vi "CLC_Gen3_L1_ComGainPhase_ENA.vi"() -> ()   [LabVIEW 2023, in "Clover_Cell.lvlib"]
uses:
  lib/CTL/Keysight_VNA.ctl
  Clover_Cell.lvlib
  lib/Keysight/Keysight.lvlib
panel:
  in  "Element Gain":i32
  in  "Waiting Time(ms)":u32=100
  in  "sParameter":i32=21
  in  "Step_Freq(GHz)":dbl=0.5 format="%#_13g"
  in  "Stop_Freq(GHz)":dbl=31.5
  in  "Start_Freq(GHz)":dbl=26.5
  in  "Polarity":u16(ring) items=["H", "V"]
  in  "TRXmode":u16(ring)=1 items=["Rx"=2, "Tx"=1]
  out "Step-2":bool
  out "PHASE 2":i32
  out "GAIN 2":i32
  out "Channel 2":i32
  out "Step-1":bool
  out "Channel":i32
  out "GAIN":i32
  out "PHASE":i32
  out "Marker_array":dbl[](array[numeric])
  out "Phase":dbl[][](graph)
  in  "FileName_Note":string
  in  "VISA resource name":refnum<visa-resource-name>="TCPIP0::192.168.100.12::inst0::INSTR"
  out "Return State":bool
  out "output cluster":T1={"address"="192.168.100.111", "remote port or service name"=5025, "timeout ms (60000)"=10000}
  out "Gain":dbl[][](graph)
  out "error out":errorcluster
  # "CLC-Gen3-L1-COMGainPhase-Sweep-ENA"
  # "Setting"
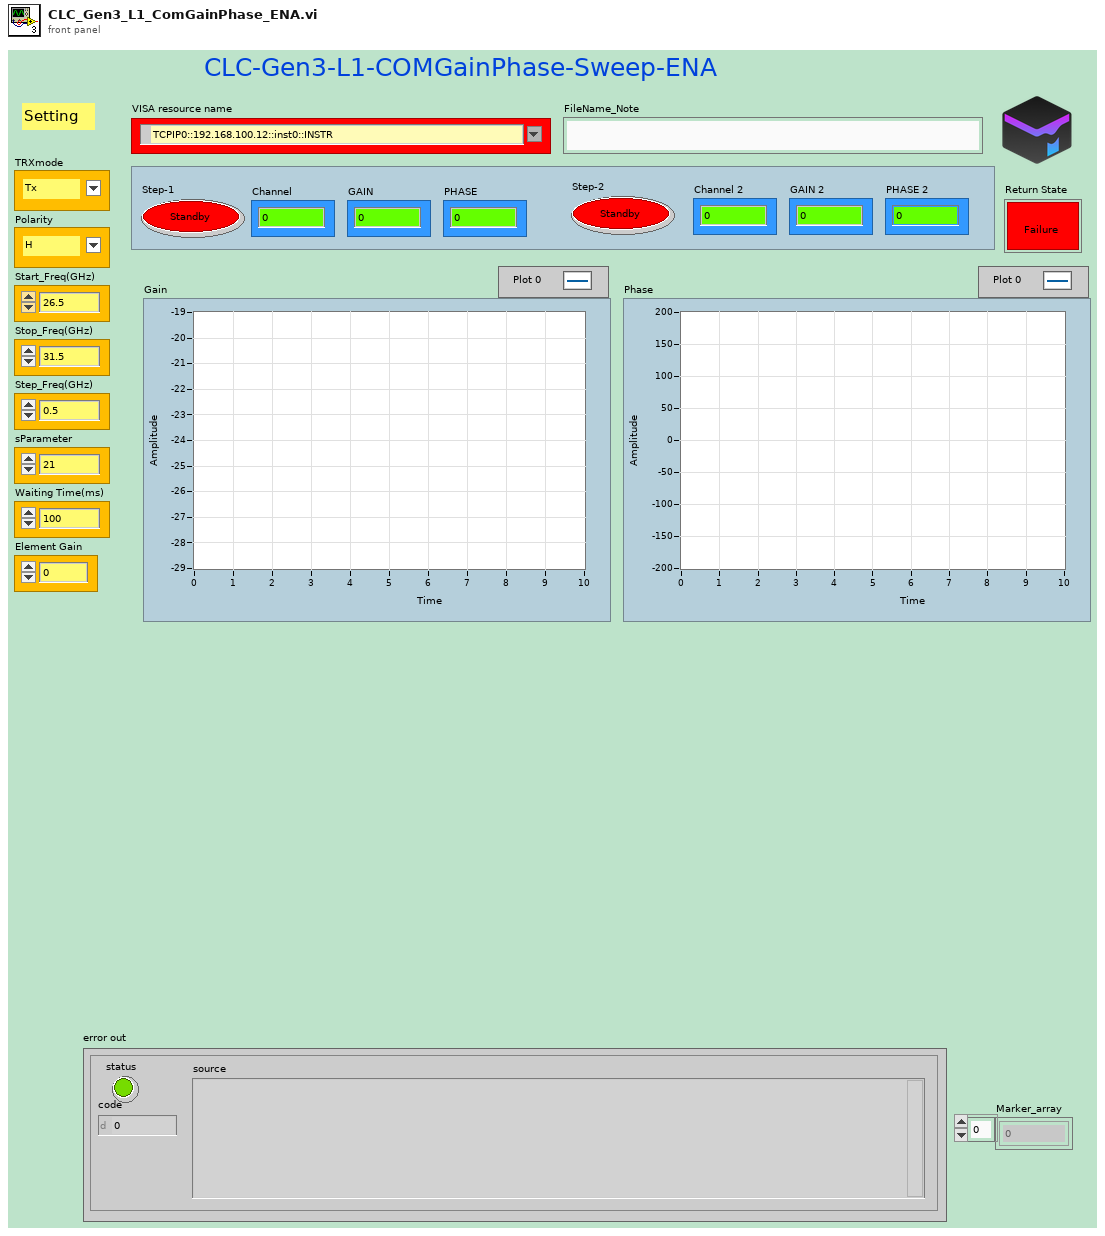
[diagram p1: front panel]
types:
  T1 = cluster{"address":string, "remote port or service name":u16, "timeout ms (60000)":i32}
  T2 = typedef "Keysight_VNA.ctl" = enum16{"Init", "queryMarker", "setSweepPoint", "setMarkerFreq", "setMeasureFormat", "setFreqStartStop", "setMarkerOnOFF", "setMarkerFormat_LOGP", "setMeasPAR_S", "setTriggerSingle", "Trigger_Save_SnP", "Trigger_Single", "Close"}
  T3 = cluster{"Mode":u16, "Polarity":u16, "CH_ON/OFF":u16, "Channel":i32, "Gain":i32, "Phase":i32}
  T4 = cluster{"setSweepPoint":i32, "Meas":i32, "Mark":i32, "Freq_GHz":dbl, "Start_Freq(GHz)":dbl, "Stop_Freq(GHz)":dbl, "sParameter":i32}
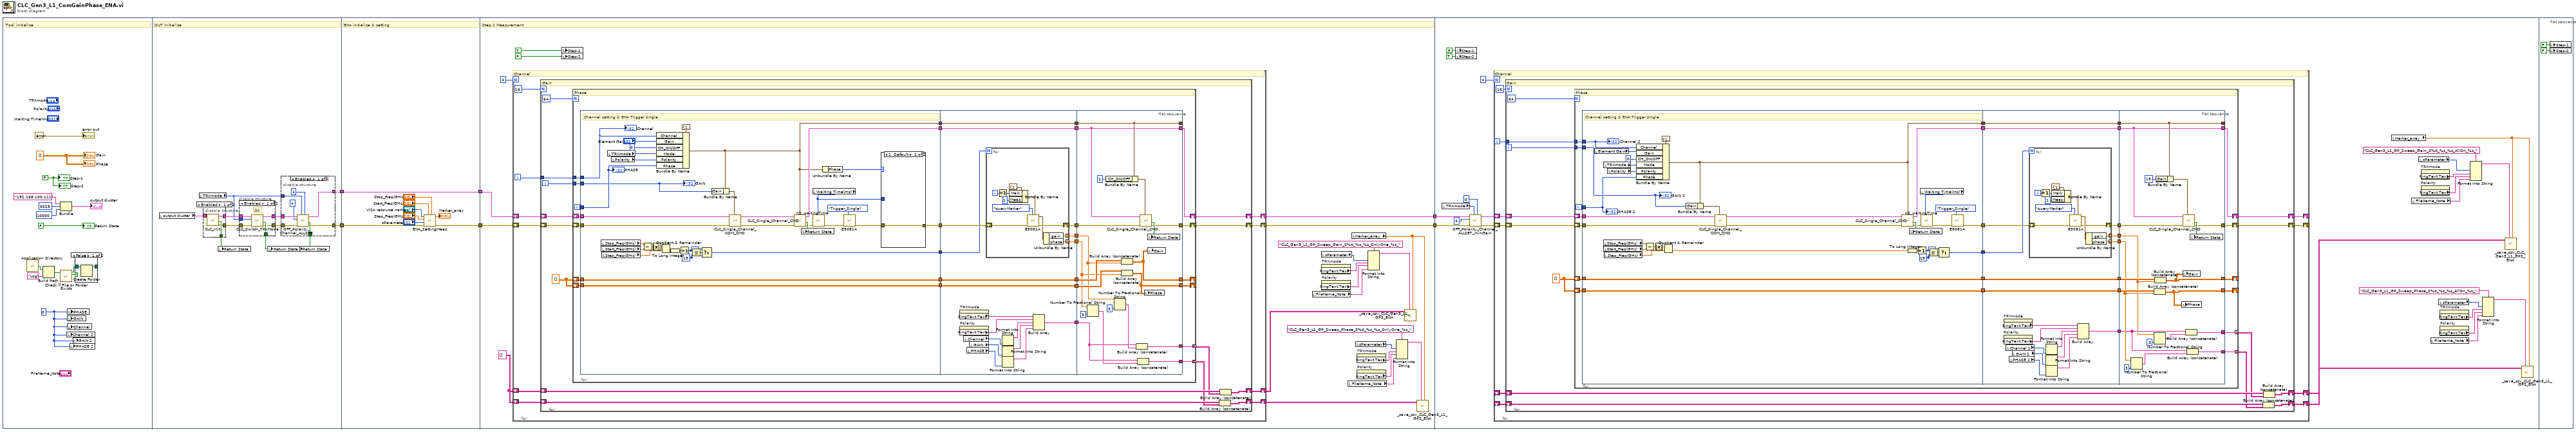
[diagram p0: block diagram]
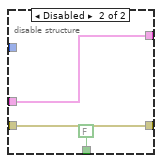
[diagram p3: hidden frame]
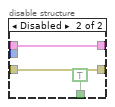
[diagram p4: hidden frame]
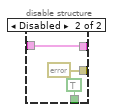
[diagram p5: hidden frame]
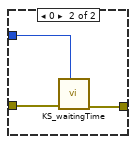
[diagram p6: hidden frame]
diagram:
  n1 = flat-sequence {
    tunnel: [w25] -> w6
    tunnel: [w29] -> w5
    tunnel: w6 -> [w70]
    tunnel: w5 -> [w63]
    tunnel: [w70] -> w4
    tunnel: [w64] -> w3
    tunnel: w4 -> [w93]
    tunnel: w3 -> [w90]
    tunnel: [w92] -> w2
    tunnel: [w91] -> w1
    tunnel: w2 -> [w254]
    tunnel: w1 -> [w255]
    frame #0 {
      w8 = FALSE ("Step-1")
      w7 = 0 ("PHASE")
      w9 = dbl[][] []
      # "Tool initialize"
      n2 = call <vilib>:"Application Directory.vi"() -> ("Application Directory"=w13:path)
      n3 = Build Path(base path=w13, name or relative path="Log") -> (appended path=w10:path)
      n4 = Bundle("address"="192.168.100.111", "remote port or service name"=u16 5025, "timeout ms (60000)"=10000) -> (→"output cluster":T1)  [unwired: 1 in]
      n5 = call <vilib>:"Check if File or Folder Exists.vi"("path"=w10) -> ("file or folder exists?"=w12:bool, "dup path"=w11:path)  [unwired: 8 in, 1 out]
      n6 = local write "Channel 2"(w7) -> ()
      n7 = local write "PHASE"(w7) -> ()
      n8 = local write "GAIN"(w7) -> ()
      n9 = local write "Channel"(w7) -> ()
      n10 = local write "PHASE 2"(w7) -> ()
      n11 = local write "GAIN 2"(w7) -> ()
      n12 = case shown="False" w12 {
        tunnel: w11 -> [w22 w23]
        tunnel: [w21 w23] -> _
        frame False {
          n13 = Create Folder(path (use dialog)=w22) -> (created path=w21:path)  [unwired: 2 in, 2 out]
        }
        frame True {
        }
      }
      "error out" <- errorcluster {"status"=FALSE, "code"=0, "source"=""} ("error out")
      "Return State" <- FALSE ("OK?")
      "Gain" <- w9
      "Phase" <- w9
      "Step-1" <- w8
      "Step-2" <- w8
    }
    frame #1 {
      # "DUT initialize"
      n14 = local read "output cluster"() -> (w34:T1)
      n15 = local read "TRXmode"() -> (w24:u16)
      n16 = disable-structure shown="Enabled" {
        disable-tunnel: w34 -> [w58 w61]
        disable-tunnel: [w57 w61] -> w33
        disable-tunnel: [w56 errorcluster {"status"=FALSE, "code"=0, "source"=""} ("error in (no error)")] -> w31
        disable-tunnel: [w55 TRUE ("OK?")] -> w26
        frame Enabled {
          n17 = call "CLC_Init.vi"("TCPIPin"=w58) -> ("error out"=w56:errorcluster, "Status"=w55:bool, "TCPIPin 2"=w57:T1)  [unwired: 8 in]
        }
        frame Disabled {
        }
      }
      n18 = local write "Return State"(w26) -> ()
      n19 = disable-structure shown="Enabled" {
        disable-tunnel: w33 -> [w51 w53]
        disable-tunnel: [w50 TRUE ("OK?")] -> w32
        disable-tunnel: w31 -> [w49 w52]
        disable-tunnel: [w48 w52] -> w30
        disable-tunnel: [w47 w53] -> w28
        disable-tunnel: w24 -> [w46 _]
        frame Enabled {
          # "OK"
          n20 = call "CLC_Switch_TRxMode.vi"("error in (no error)"=w49, "Text Ring"=w46, "TCPIPin"=w51) -> ("error out"=w48:errorcluster, "OK?"=w50:bool, "TCPIPin 2"=w47:T1)  [unwired: 6 in]
        }
        frame Disabled {
        }
      }
      n21 = local write "Return State"(w32) -> ()
      n22 = disable-structure shown="Enabled" {
        disable-tunnel: w30 -> [w42 w44]
        disable-tunnel: [w41 w44] -> w29
        disable-tunnel: w28 -> [w40 w43]
        disable-tunnel: [w39 FALSE ("OK?")] -> w27
        disable-tunnel: w24 -> [w37 _]
        disable-tunnel: [w35 w43] -> w25
        frame Enabled {
          n23 = call "OFF_Polarity_Channel_ALLSET.vi"("CH_ON:0/OFF:1"=u16 1, "Mode"=w37, "error in"=w42, "Channel"=4, "TCPIPin"=w40) -> ("error out"=w41:errorcluster, "OK?"=w39:bool, "TCPIPout"=w35:T1)  [unwired: 4 in]
        }
        frame Disabled {
        }
      }
      n24 = local write "Return State"(w27) -> ()
    }
    frame #2 {
      # "ENA initialize & setting"
      n25 = call "ENA_SettingMeas.vi"("Stop_Freq(GHz)"="Stop_Freq(GHz)", "Start_Freq(GHz)"="Start_Freq(GHz)", "error in"=w63, "sParameter"="sParameter", "Step_Freq(GHz)"="Step_Freq(GHz)", "VISA IN"="VISA resource name") -> ("error out"=w64:errorcluster, "Marker_array"=→"Marker_array":dbl[])  [unwired: 4 in]
    }
    frame #3 {
      w88 = string[][] []
      # "Step.1 Measurement"
      n26 = for {
        N: 4 -> [_]
        shift-right: [w102] -> w92
        shift-left: w93 -> [w103]
        shift-right: [w101] -> w91
        shift-left: w90 -> [w100]
        shift-right: [w95] -> w87
        shift-left: w88 -> [w97]
        shift-right: [w94] -> w86
        shift-left: w88 -> [w96]
        i -> [w98]
        # "Channel"
        n27 = for {
          N: 16 -> [_]
          shift-right: [w116] -> w102
          shift-left: w103 -> [w117]
          shift-right: [w115] -> w101
          shift-left: w100 -> [w114]
          tunnel: w98 -> [w112]
          shift-right: [w106] -> w95
          shift-left: w97 -> [w110]
          shift-right: [w105] -> w94
          shift-left: w96 -> [w109]
          i -> [w111]
          w104 = dbl[][] []
          # "Gain"
          n28 = for {
            N: 64 -> [_]
            shift-right: [w132] -> w116
            shift-left: w117 -> [w144]
            shift-right: [w131] -> w115
            shift-left: w114 -> [w143]
            tunnel: w112 -> [w142]
            tunnel: w111 -> [w141]
            tunnel: [w127] -> w108 mode=indexing
            tunnel: [w126] -> w107 mode=indexing
            shift-right: [w119] -> _
            shift-left: w104 -> [w123]
            shift-right: [w118] -> _
            shift-left: w104 -> [w120]
            i -> [w140]
            # "Phase"
            n29 = flat-sequence {
              tunnel: w144 -> [w154]
              tunnel: w143 -> [w155]
              tunnel: w142 -> [w178]
              tunnel: w141 -> [w151]
              tunnel: w140 -> [w171]
              tunnel: [w148] -> w139
              tunnel: [w160] -> w138
              tunnel: [w146] -> w137
              tunnel: [w159] -> w136
              tunnel: [w158] -> w124
              tunnel: w123 -> [w158]
              tunnel: [w157] -> w121
              tunnel: w120 -> [w157]
              tunnel: w139 -> [w201]
              tunnel: w138 -> [w200]
              tunnel: w137 -> [w199]
              tunnel: w136 -> [w198]
              tunnel: [w202] -> w135
              tunnel: [w200] -> w134
              tunnel: [w199] -> w133
              tunnel: [w197] -> w130
              tunnel: [w196] -> w129
              tunnel: [w187] -> w128
              tunnel: [w186] -> w125
              tunnel: w124 -> [w186]
              tunnel: [w185] -> w122
              tunnel: w121 -> [w185]
              tunnel: [w230] -> _
              tunnel: [w227] -> w132
              tunnel: [w232] -> w131
              tunnel: w135 -> [w231]
              tunnel: w134 -> [w227]
              tunnel: w133 -> [w230]
              tunnel: w130 -> [w217]
              tunnel: w129 -> [w216]
              tunnel: w128 -> [w223]
              tunnel: [w221] -> w127
              tunnel: [w220] -> w126
              tunnel: w125 -> [w219]
              tunnel: w122 -> [w218]
              tunnel: [w215] -> w119
              tunnel: [w214] -> w118
              frame #0 {
                w170 = 15 ("y")
                # "Channel setting & ENA Trigger single"
                n30 = local read "Stop_Freq(GHz)"() -> (w163:dbl)
                n31 = local read "Start_Freq(GHz)"() -> (w162:dbl)
                n32 = local read "Step_Freq(GHz)"() -> (w161:dbl)
                n33 = local read "TRXmode"() -> (w176:u16)
                n34 = local read "Polarity"() -> (w177:u16)
                n35 = Subtract(x=w163, y=w162) -> (x-y=w169:dbl)
                n36 = Absolute Value(x=w169) -> (abs(x)=w168:dbl)
                n37 = Bundle By Name(cluster=T3 {"Mode"=1, "Polarity"=1, "CH_ON/OFF"=1, "Channel"=0, "Gain"=0, "Phase"=0} ("Channel params"), "Channel"=w178, "Gain"="Element Gain", "CH_ON/OFF"=u16 0, "Mode"=w176, "Polarity"=w177, "Phase"=w171) -> (w146:T3)
                n38 = Quotient & Remainder(x=w168, y=w161) -> (floor(x/y)=w167:dbl)  [unwired: 1 out]
                n39 = To Long Integer(number=w167) -> (32bit integer=w166:i32)
                n40 = Increment(x=w166) -> (x+1=w164:i32)
                n41 = Less Or Equal?(x=w164, y=w170) -> (x <= y?=w165:bool)
                n42 = Select(t=w164, s=w165, f=w170) -> (s? t:f=w159:i32)
                n43 = Bundle By Name(cluster=w146, "Gain"=w151) -> (w150:T3)
                n44 = call "CLC_Single_Channel_COM_CMD.vi"("Channel params"=w150, "error in"=w155, "TCPIPin"=w154) -> ("error out"=w156:errorcluster, "TCPIPout"=w153:T1)  [unwired: 6 in, 1 out]
                n45 = call "CLC_Single_Channel_CMD.vi"("Channel params"=w146, "error in"=w156, "TCPIPin"=w153) -> ("error out"=w175:errorcluster, "OK?"=w179:bool, "TCPIPout"=w160:T1)  [unwired: 6 in]
                n46 = local write "Return State"(w179) -> ()
                n47 = local read "Waiting Time(ms)"() -> (w147:u32)
                n48 = call "KS_waitingTime.vi"("Waiting Time(ms)"=w147, "error in"=w175) -> ("error out"=w173:errorcluster)  [unwired: 9 in]
                n49 = Unbundle By Name(w146) -> ("Phase"=w145:i32)
                n50 = call "E5081A.vi"("Function_VNA"=Keysight_VNA."Trigger_Single", "error in"=w173) -> ("error out"=w149:errorcluster)  [unwired: 8 in, 1 out]
                n51 = case shown="1, Default" w145 {
                  tunnel: w149 -> [w181 w184]
                  tunnel: [w181 w183] -> w148
                  tunnel: w147 -> [_ w182]
                  frame 1, Default {
                  }
                  frame 0 {
                    n52 = call "KS_waitingTime.vi"("Waiting Time(ms)"=w182, "error in"=w184) -> ("error out"=w183:errorcluster)  [unwired: 9 in]
                  }
                }
                "PHASE" <- w171
                "GAIN" <- w151
                "Channel" <- w178
              }
              frame #1 {
                n53 = property on="TRXmode" class="Ring (strict)"() -> ("RingText.Text"=w192:string)  [unwired: 2 in, 2 out]
                n54 = property on="Polarity" class="Ring (strict)"() -> ("RingText.Text"=w191:string)  [unwired: 2 in, 2 out]
                n55 = local read "Channel"() -> (w195:i32)
                n56 = local read "PHASE"() -> (w193:i32)
                n57 = local read "GAIN"() -> (w194:i32)
                n58 = for {
                  N: w198 -> [_]
                  shift-right: [w212] -> w202
                  shift-left: w201 -> [w213]
                  tunnel: [w204] -> w197 mode=indexing
                  tunnel: [w203] -> w196 mode=indexing
                  i -> [w209]
                  n59 = Increment(x=w209) -> (x+1=w207:i32)
                  n60 = Bundle By Name(cluster=T4 {"setSweepPoint"=11, "Meas"=1, "Mark"=0, "Freq_GHz"=0.0, "Start_Freq(GHz)"=0.0, "Stop_Freq(GHz)"=0.0, "sParameter"=1} ("Input"), "Mark"=w207, "Meas"=1) -> (w206:T4)
                  n61 = call "E5081A.vi"("Input"=w206, "Function_VNA"=Keysight_VNA."queryMarker", "error in"=w213) -> ("error out"=w212:errorcluster, "queryMarker"=w205:cluster{"gain":dbl, "phase":dbl})  [unwired: 7 in]
                  n62 = Unbundle By Name(w205) -> ("gain"=w204:dbl, "phase"=w203:dbl)
                }
                n63 = Format Into String(w195) -> (resulting string=w190:string)  [unwired: 3 in, 1 out]
                n64 = Format Into String(w194) -> (resulting string=w189:string)  [unwired: 3 in, 1 out]
                n65 = Format Into String(w193) -> (resulting string=w188:string)  [unwired: 3 in, 1 out]
                n66 = Build Array(w192, w191, w190, w189, w188) -> (w187:string[])
              }
              frame #2 {
                n67 = Number To Fractional String(number=w216, precision (6)=i16 3) -> (F-format string=w222:string[])  [unwired: 2 in]
                n68 = Bundle By Name(cluster=w230, "CH_ON/OFF"=u16 1) -> (w228:T3)
                n69 = Number To Fractional String(number=w217, precision (6)=i16 3) -> (F-format string=w224:string[])  [unwired: 2 in]
                n70 = Build Array (concatenate)(w218, w216) -> (w214:dbl[][])
                n71 = Build Array (concatenate)(w219, w217) -> (w215:dbl[][])
                n72 = Build Array (concatenate)(w223, w224) -> (w221:string[])
                n73 = Build Array (concatenate)(w223, w222) -> (w220:string[])
                n74 = call "CLC_Single_Channel_CMD.vi"("Channel params"=w228, "error in"=w231, "TCPIPin"=w227) -> ("error out"=w232:errorcluster, "OK?"=w233:bool)  [unwired: 6 in, 1 out]
                n75 = local write "Phase"(w214) -> ()
                n76 = local write "Return State"(w233) -> ()
                n77 = local write "Gain"(w215) -> ()
              }
            }
          }
          n78 = Build Array (concatenate)(w109, w107) -> (w105:string[][])
          n79 = Build Array (concatenate)(w110, w108) -> (w106:string[][])
        }
      }
      n80 = local write "Step-1"(TRUE ("Step-1")) -> ()
      n81 = local write "Step-2"(FALSE ("Step-2")) -> ()
      n82 = local read "FileName_Note"() -> (w74:string)
      n83 = local read "sParameter"() -> (w77:i32)
      n84 = property on="TRXmode" class="Ring (strict)"() -> ("RingText.Text"=w76:string)  [unwired: 2 in, 2 out]
      n85 = property on="Polarity" class="Ring (strict)"() -> ("RingText.Text"=w75:string)  [unwired: 2 in, 2 out]
      n86 = local read "FileName_Note"() -> (w71:string)
      n87 = local read "Marker_array"() -> (w85:dbl[])
      n88 = local read "sParameter"() -> (w82:i32)
      n89 = property on="TRXmode" class="Ring (strict)"() -> ("RingText.Text"=w73:string)  [unwired: 2 in, 2 out]
      n90 = property on="Polarity" class="Ring (strict)"() -> ("RingText.Text"=w72:string)  [unwired: 2 in, 2 out]
      n91 = Format Into String(format string="CLC_Gen3_L1_GP_Sweep_Gain_S%d_%s_%s_OnlyOne_%s_" ("NoteName"), w77, w76, w75, w74) -> (resulting string=w83:string)  [unwired: 2 in, 1 out]
      n92 = Format Into String(format string="CLC_Gen3_L1_GP_Sweep_Phase_S%d_%s_%s_OnlyOne_%s_" ("NoteName"), w82, w73, w72, w71) -> (resulting string=w80:string)  [unwired: 2 in, 1 out]
      n93 = call "_save_csv_CLC_Gen3_L1_GPS_ENA.vi"("Marker_array"=w85, "NoteName"=w83, "array in"=w87) -> ()  [unwired: 8 in, 1 out]
      n94 = call "_save_csv_CLC_Gen3_L1_GPS_ENA.vi"("Marker_array"=w85, "NoteName"=w80, "array in"=w86) -> ()  [unwired: 8 in, 1 out]
    }
    frame #4 {
      n95 = local read "TRXmode"() -> (w252:u16)
      n96 = local write "Step-1"(FALSE ("Step-1")) -> ()
      n97 = local write "Step-2"(TRUE ("Step-2")) -> ()
      n98 = call "OFF_Polarity_Channel_ALLSET_minGain.vi"("CH_ON:0/OFF:1"=u16 0, "Mode"=w252, "error in"=w255, "Channel"=4, "TCPIPin"=w254) -> ("error out"=w256:errorcluster, "TCPIPout"=w257:T1)  [unwired: 4 in, 1 out]
      n99 = for {
        N: 4 -> [_]
        shift-right: [w267] -> _
        shift-left: w257 -> [w268]
        shift-right: [w266] -> _
        shift-left: w256 -> [w265]
        shift-right: [w260] -> w244
        shift-left: _ -> [w262]
        shift-right: [w259] -> w243
        shift-left: _ -> [w261]
        i -> [w263]
        # "Channel"
        n100 = for {
          N: 16 -> [_]
          shift-right: [w281] -> w267
          shift-left: w268 -> [w282]
          shift-right: [w280] -> w266
          shift-left: w265 -> [w279]
          tunnel: w263 -> [w277]
          shift-right: [w271] -> w260
          shift-left: w262 -> [w275]
          shift-right: [w270] -> w259
          shift-left: w261 -> [w274]
          i -> [w276]
          w269 = dbl[][] []
          # "Gain"
          n101 = for {
            N: 64 -> [_]
            shift-right: [w297] -> w281
            shift-left: w282 -> [w309]
            shift-right: [w296] -> w280
            shift-left: w279 -> [w308]
            tunnel: w277 -> [w307]
            tunnel: w276 -> [w306]
            tunnel: [w292] -> w273 mode=indexing
            tunnel: [w291] -> w272 mode=indexing
            shift-right: [w284] -> _
            shift-left: w269 -> [w288]
            shift-right: [w283] -> _
            shift-left: w269 -> [w285]
            i -> [w305]
            # "Phase"
            n102 = flat-sequence {
              tunnel: w309 -> [w314]
              tunnel: w308 -> [w316]
              tunnel: w307 -> [w341]
              tunnel: w306 -> [w312]
              tunnel: w305 -> [w333]
              tunnel: [w335] -> w304
              tunnel: [w322] -> w303
              tunnel: [w311] -> w302
              tunnel: [w321] -> w301
              tunnel: [w319] -> w289
              tunnel: w288 -> [w319]
              tunnel: [w318] -> w286
              tunnel: w285 -> [w318]
              tunnel: w304 -> [w360]
              tunnel: w303 -> [w359]
              tunnel: w302 -> [w358]
              tunnel: w301 -> [w357]
              tunnel: [w361] -> w300
              tunnel: [w359] -> w299
              tunnel: [w358] -> w298
              tunnel: [w356] -> w295
              tunnel: [w355] -> w294
              tunnel: [w346] -> w293
              tunnel: [w345] -> w290
              tunnel: w289 -> [w345]
              tunnel: [w344] -> w287
              tunnel: w286 -> [w344]
              tunnel: [w389] -> _
              tunnel: [w387] -> w297
              tunnel: [w391] -> w296
              tunnel: w300 -> [w390]
              tunnel: w299 -> [w387]
              tunnel: w298 -> [w389]
              tunnel: w295 -> [w376]
              tunnel: w294 -> [w373]
              tunnel: w293 -> [w383]
              tunnel: [w381] -> w292
              tunnel: [w380] -> w291
              tunnel: w290 -> [w378]
              tunnel: w287 -> [w377]
              tunnel: [w375] -> w284
              tunnel: [w374] -> w283
              frame #0 {
                w332 = 15 ("y")
                # "Channel setting & ENA Trigger single"
                n103 = local read "Element Gain"() -> (w313:i32)
                n104 = local read "TRXmode"() -> (w339:u16)
                n105 = local read "Stop_Freq(GHz)"() -> (w325:dbl)
                n106 = local read "Start_Freq(GHz)"() -> (w324:dbl)
                n107 = local read "Step_Freq(GHz)"() -> (w323:dbl)
                n108 = local read "Polarity"() -> (w340:u16)
                n109 = Bundle By Name(cluster=T3 {"Mode"=1, "Polarity"=1, "CH_ON/OFF"=1, "Channel"=0, "Gain"=0, "Phase"=0} ("Channel params"), "Channel"=w341, "Gain"=w313, "CH_ON/OFF"=u16 0, "Mode"=w339, "Polarity"=w340, "Phase"=w333) -> (w311:T3)
                n110 = Subtract(x=w325, y=w324) -> (x-y=w331:dbl)
                n111 = Absolute Value(x=w331) -> (abs(x)=w330:dbl)
                n112 = Quotient & Remainder(x=w330, y=w323) -> (floor(x/y)=w329:dbl)  [unwired: 1 out]
                n113 = Bundle By Name(cluster=w311, "Gain"=w312) -> (w310:T3)
                n114 = call "CLC_Single_Channel_COM_CMD.vi"("Channel params"=w310, "error in"=w316, "TCPIPin"=w314) -> ("error out"=w317:errorcluster, "TCPIPout"=w315:T1)  [unwired: 6 in, 1 out]
                n115 = call "CLC_Single_Channel_CMD.vi"("Channel params"=w311, "error in"=w317, "TCPIPin"=w315) -> ("error out"=w338:errorcluster, "OK?"=w342:bool, "TCPIPout"=w322:T1)  [unwired: 6 in]
                n116 = To Long Integer(number=w329) -> (32bit integer=w328:i32)
                n117 = local write "Return State"(w342) -> ()
                n118 = Increment(x=w328) -> (x+1=w326:i32)
                n119 = local read "Waiting Time(ms)"() -> (w320:u32)
                n120 = call "KS_waitingTime.vi"("Waiting Time(ms)"=w320, "error in"=w338) -> ("error out"=w336:errorcluster)  [unwired: 9 in]
                n121 = Less Or Equal?(x=w326, y=w332) -> (x <= y?=w327:bool)
                n122 = Select(t=w326, s=w327, f=w332) -> (s? t:f=w321:i32)
                n123 = call "E5081A.vi"("Function_VNA"=Keysight_VNA."Trigger_Single", "error in"=w336) -> ("error out"=w335:errorcluster)  [unwired: 8 in, 1 out]
                "PHASE 2" <- w333
                "GAIN 2" <- w312
                "Channel 2" <- w341
              }
              frame #1 {
                n124 = property on="TRXmode" class="Ring (strict)"() -> ("RingText.Text"=w351:string)  [unwired: 2 in, 2 out]
                n125 = property on="Polarity" class="Ring (strict)"() -> ("RingText.Text"=w350:string)  [unwired: 2 in, 2 out]
                n126 = local read "Channel 2"() -> (w354:i32)
                n127 = local read "PHASE 2"() -> (w352:i32)
                n128 = local read "GAIN 2"() -> (w353:i32)
                n129 = for {
                  N: w357 -> [_]
                  shift-right: [w371] -> w361
                  shift-left: w360 -> [w372]
                  tunnel: [w363] -> w356 mode=indexing
                  tunnel: [w362] -> w355 mode=indexing
                  i -> [w368]
                  n130 = Increment(x=w368) -> (x+1=w366:i32)
                  n131 = Bundle By Name(cluster=T4 {"setSweepPoint"=11, "Meas"=1, "Mark"=0, "Freq_GHz"=0.0, "Start_Freq(GHz)"=0.0, "Stop_Freq(GHz)"=0.0, "sParameter"=1} ("Input"), "Mark"=w366, "Meas"=1) -> (w365:T4)
                  n132 = call "E5081A.vi"("Input"=w365, "Function_VNA"=Keysight_VNA."queryMarker", "error in"=w372) -> ("error out"=w371:errorcluster, "queryMarker"=w364:cluster{"gain":dbl, "phase":dbl})  [unwired: 7 in]
                  n133 = Unbundle By Name(w364) -> ("gain"=w363:dbl, "phase"=w362:dbl)
                }
                n134 = Format Into String(w354) -> (resulting string=w349:string)  [unwired: 3 in, 1 out]
                n135 = Format Into String(w353) -> (resulting string=w348:string)  [unwired: 3 in, 1 out]
                n136 = Format Into String(w352) -> (resulting string=w347:string)  [unwired: 3 in, 1 out]
                n137 = Build Array(w351, w350, w349, w348, w347) -> (w346:string[])
              }
              frame #2 {
                n138 = Number To Fractional String(number=w373, precision (6)=i16 3) -> (F-format string=w382:string[])  [unwired: 2 in]
                n139 = Build Array (concatenate)(w377, w373) -> (w374:dbl[][])
                n140 = Number To Fractional String(number=w376, precision (6)=i16 3) -> (F-format string=w384:string[])  [unwired: 2 in]
                n141 = Build Array (concatenate)(w378, w376) -> (w375:dbl[][])
                n142 = Bundle By Name(cluster=w389, "Gain"=15) -> (w388:T3)
                n143 = local write "Phase"(w374) -> ()
                n144 = call "CLC_Single_Channel_CMD.vi"("Channel params"=w388, "error in"=w390, "TCPIPin"=w387) -> ("error out"=w391:errorcluster, "OK?"=w392:bool)  [unwired: 6 in, 1 out]
                n145 = local write "Gain"(w375) -> ()
                n146 = Build Array (concatenate)(w383, w384) -> (w381:string[])
                n147 = Build Array (concatenate)(w383, w382) -> (w380:string[])
                n148 = local write "Return State"(w392) -> ()
              }
            }
          }
          n149 = Build Array (concatenate)(w274, w272) -> (w270:string[][])
          n150 = Build Array (concatenate)(w275, w273) -> (w271:string[][])
        }
      }
      n151 = local read "Marker_array"() -> (w250:dbl[])
      n152 = local read "FileName_Note"() -> (w237:string)
      n153 = local read "sParameter"() -> (w240:i32)
      n154 = property on="TRXmode" class="Ring (strict)"() -> ("RingText.Text"=w239:string)  [unwired: 2 in, 2 out]
      n155 = property on="Polarity" class="Ring (strict)"() -> ("RingText.Text"=w238:string)  [unwired: 2 in, 2 out]
      n156 = local read "FileName_Note"() -> (w234:string)
      n157 = local read "sParameter"() -> (w248:i32)
      n158 = property on="TRXmode" class="Ring (strict)"() -> ("RingText.Text"=w236:string)  [unwired: 2 in, 2 out]
      n159 = property on="Polarity" class="Ring (strict)"() -> ("RingText.Text"=w235:string)  [unwired: 2 in, 2 out]
      n160 = Format Into String(format string="CLC_Gen3_L1_GP_Sweep_Gain_S%d_%s_%s_AllOn_%s_" ("NoteName"), w240, w239, w238, w237) -> (resulting string=w249:string)  [unwired: 2 in, 1 out]
      n161 = Format Into String(format string="CLC_Gen3_L1_GP_Sweep_Phase_S%d_%s_%s_AllOn_%s_" ("NoteName"), w248, w236, w235, w234) -> (resulting string=w247:string)  [unwired: 2 in, 1 out]
      n162 = call "_save_csv_CLC_Gen3_L1_GPS_ENA.vi"("Marker_array"=w250, "NoteName"=w249, "array in"=w244) -> ()  [unwired: 8 in, 1 out]
      n163 = call "_save_csv_CLC_Gen3_L1_GPS_ENA.vi"("Marker_array"=w250, "NoteName"=w247, "array in"=w243) -> ()  [unwired: 8 in, 1 out]
    }
    frame #5 {
      n164 = local write "Step-1"(FALSE ("Step-1")) -> ()
      n165 = local write "Step-2"(FALSE ("Step-2")) -> ()
    }
  }
